vi "StringFormatGlobals.vi"() -> ()   [LabVIEW 2023]
doc: "Contains Format Strings"
panel:
  in  "XYposition WinSize":cluster{"Width":i32, "Height":i32}={"Width"=105, "Height"=50}
  in  "XYmeasure WinSize":cluster{"Width":i32, "Height":i32}={"Width"=160, "Height"=32}
  in  "Line WinSize":cluster{"Width":i32, "Height":i32}={"Width"=135, "Height"=50}
  in  "Point WinSize":cluster{"Width":i32, "Height":i32}={"Width"=102, "Height"=50}
  out "XYPosition BG Image":picture
  out "XYMeasure BG Image":picture
  out "Line BG image":picture
  out "Point BG Image":picture
  in  "XYposition Display format":string="x=%6.3f [%d]\\ny=%6.3f\\nf(x)=%f"
  in  "XYposition format read":string="xyposition X=%f [%d]\\nY=%f [%d]\\nZ=%f"
  in  "XYposition format write":string="xyposition X=%f [%d]\\nY=%f [%d]\\nZ=%f"
  in  "XYmeasure Display Format":string="   %6.3f      %6.3f\n   %6.3f      %6.3f"
  in  "XYmeasure Format write":string="xymeasure (%f,%f) (%f,%f) [%d,%d] [%d,%d]"
  in  "XYmeasure format read":string="xymeasure (%f,%f) (%f,%f) [%d,%d] [%d,%d]"
  in  "Point Display format":string="X=%6.3f [%d]\\nY=%6.3f [%d]\\nZ=%f"
  in  "Point format read":string="position X=%f [%d]\\nY=%f [%d]\\nZ=%f"
  in  "Point format write":string="position X=%f [%d]\\nY=%f [%d]\\nZ=%f"
  in  "Line Display Format":string="P1=(%6.3f,%6.3f)\nP2=(%6.3f,%6.3f)\nL=%5.3f A=%7.2f°"
  in  "Line Format write":string="line (%f,%f) (%f,%f) [%d,%d] [%d,%d]"
  in  "Line format read":string="line (%f,%f) (%f,%f) [%d,%d] [%d,%d]"
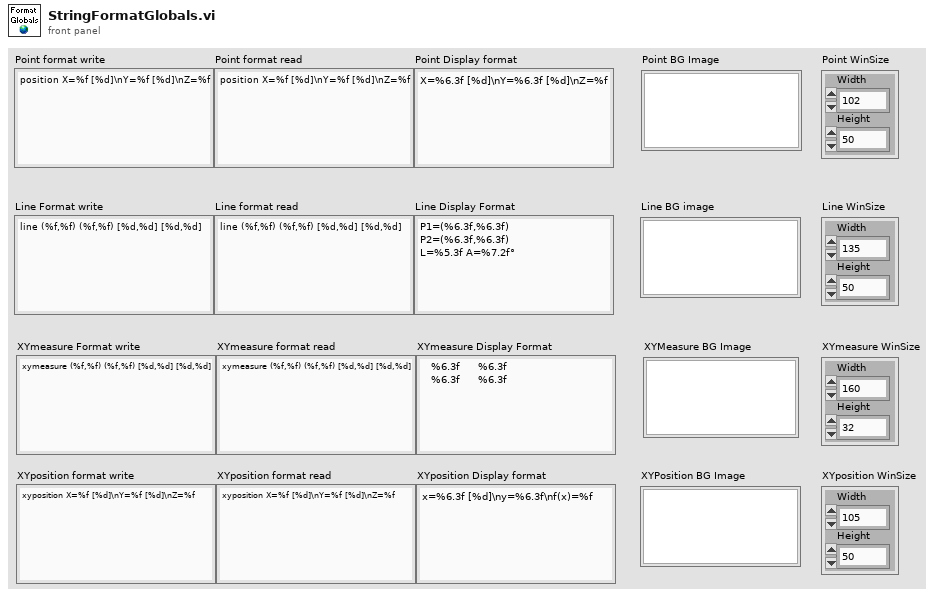
[diagram p1: front panel]
diagram:
